vi "Laser-Main-2018-06-18.vi"() -> ()   [LabVIEW 2013]
doc: "Use this template to build a user interface event handler design pattern. Use this pattern for dialog boxes and other user interfaces. You also can create and execute user-defined events that the VI can handle the same way as user interface events."
uses:
  <vilib>/Instr/_visa.llb/VISA Configure Serial Port (Instr).vi
panel:
  out "hex integer string 2":string
  out "EnergyCommand 2":string
  in  "SetTrans 2":i16=1 min=0 max=100
  in  "OFF_Laser":bool
  out "Energy":string
  out "ReturnState":string
  in  "ShutDownSystem":bool
  out "ReturnShortState":string
  out "ShortState":string
  out "LaserState":bool[](array[boolean])
  out "hex integer string":string
  out "EnergyCommand":string
  out "HVCommand":string
  out "FreqCommand":string
  in  "SetTrans":i16=1 min=0 max=100
  in  "LaserHV":u8=20
  in  "LaserFreq":u8=60
  out "LaserEnergy uJ":dbl
  in  "ComForLaser":refnum<visa-resource-name>="COM3"
  in  "Serial Settings":T1={"baud rate"=9600, "data bits"=8, "parity"=enum."None", "stop bits"=10, "flow control"=0} {"flow control" items=["None"=0, "XON/XOFF"=1, "RTS/CTS"=2, "DTR/DSR"=4]; "stop bits" items=["1.0"=10, "1.5"=15, "2.0"=20]; "data bits" min=5 max=8 step=1; "baud rate" items=["75"=75, "110"=110, "134"=134, "150"=150, "300"=300, "600"=600, "1200"=1200, "1800"=1800, "2400"=2400, "4800"=4800, "7200"=7200, "9600"=9600, "14400"=14400, "19200"=19200, "28800"=28800, "38400"=38400, "56000"=56000, "57600"=57600, "115200"=115200, "128000"=128000, "230400"=230400]}
  in  "Stop_Laser":bool
  in  "Start_Laser":bool
  # "连接"
  # "待机"
  # "发射"
  # "内存"
  # "测能"
  # "温警"
  # "静态"
  # "操作"
  # "将激光能量设置改成激光光栅设置"
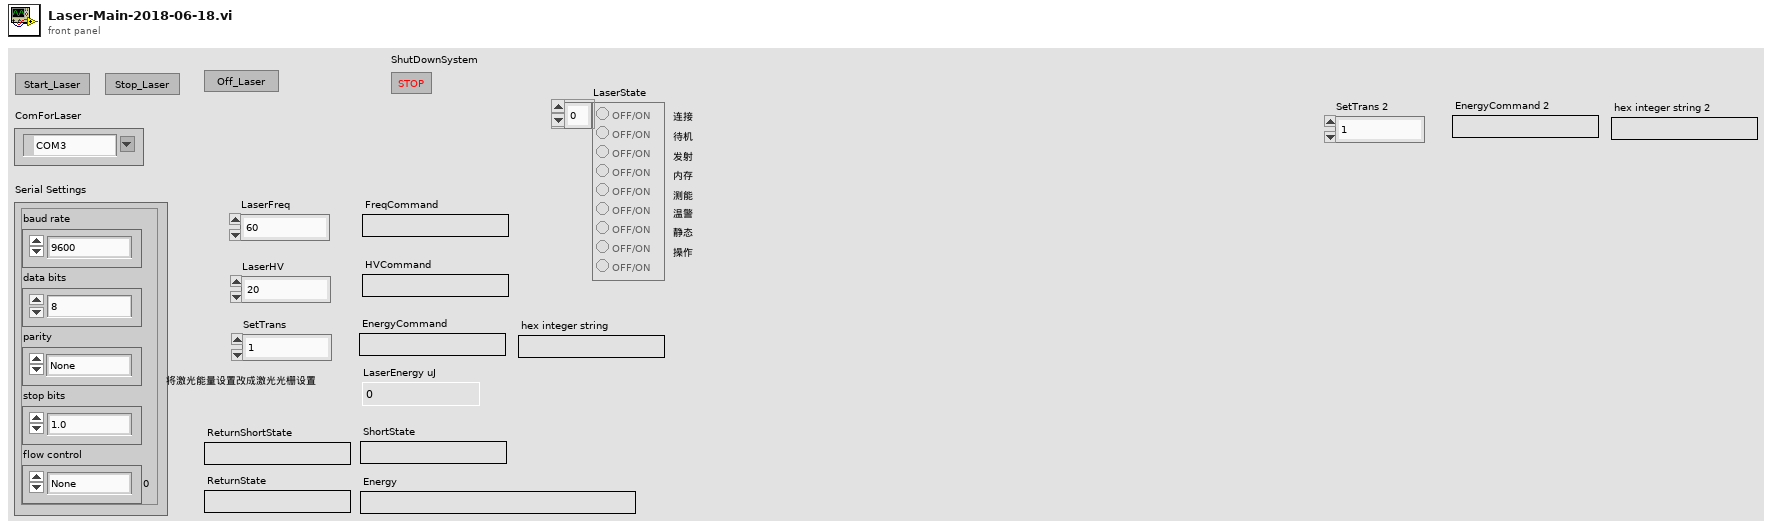
[diagram p1: front panel]
types:
  T1 = cluster{"baud rate":u32, "data bits":u16, "parity":enum16{"None", "Odd", "Even", "Mark", "Space"}, "stop bits":u16, "flow control":u16}
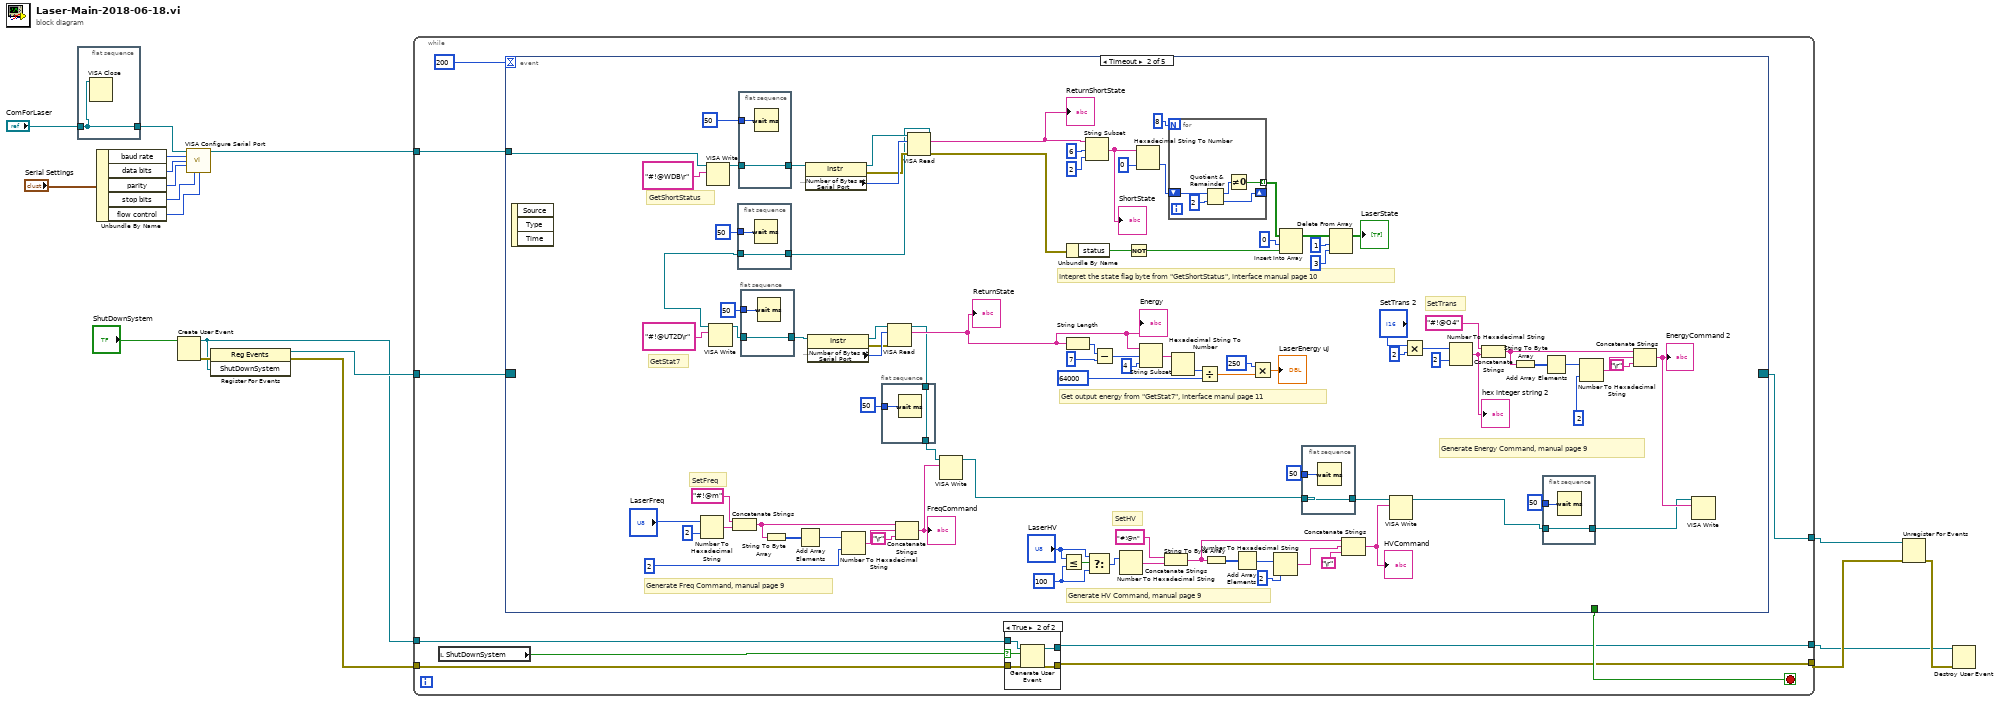
[diagram p0: block diagram]
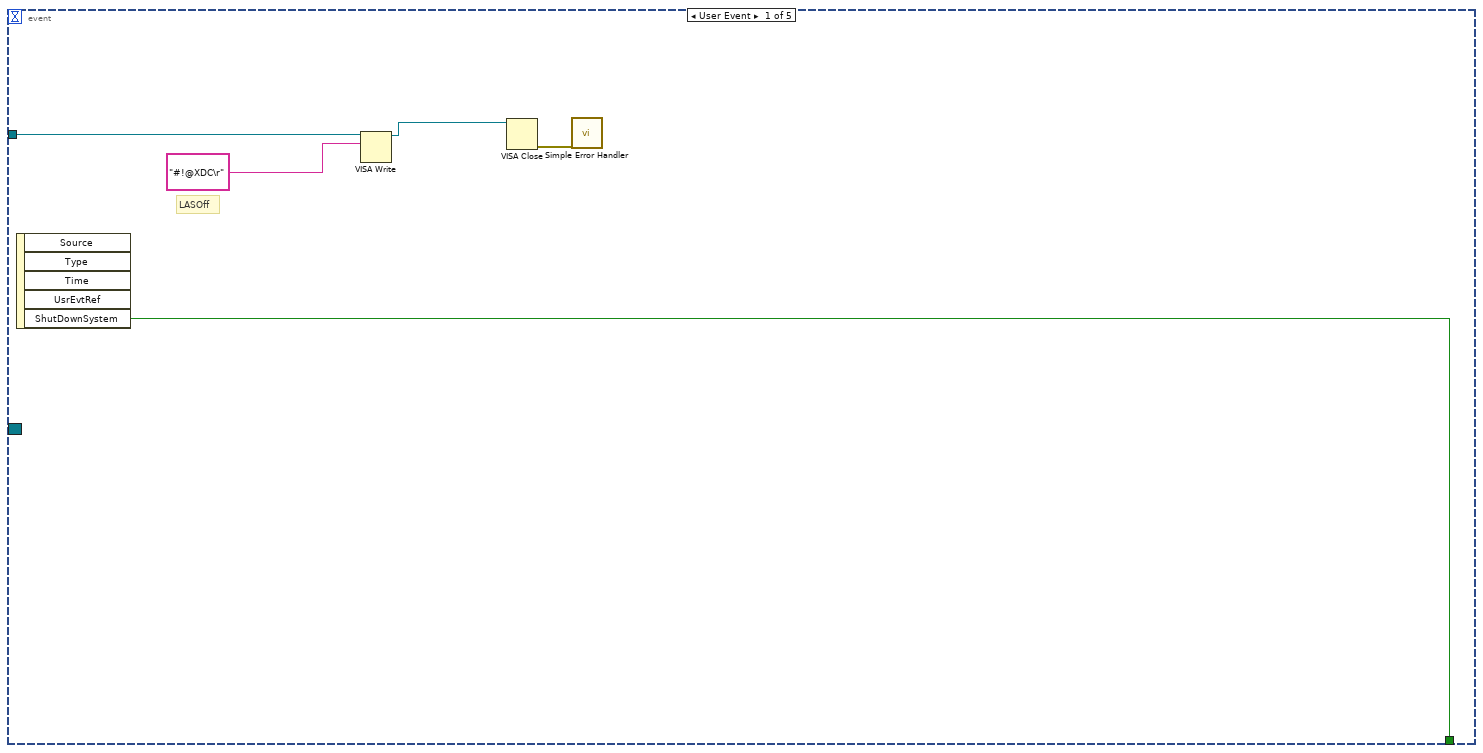
[diagram p3: hidden frame]
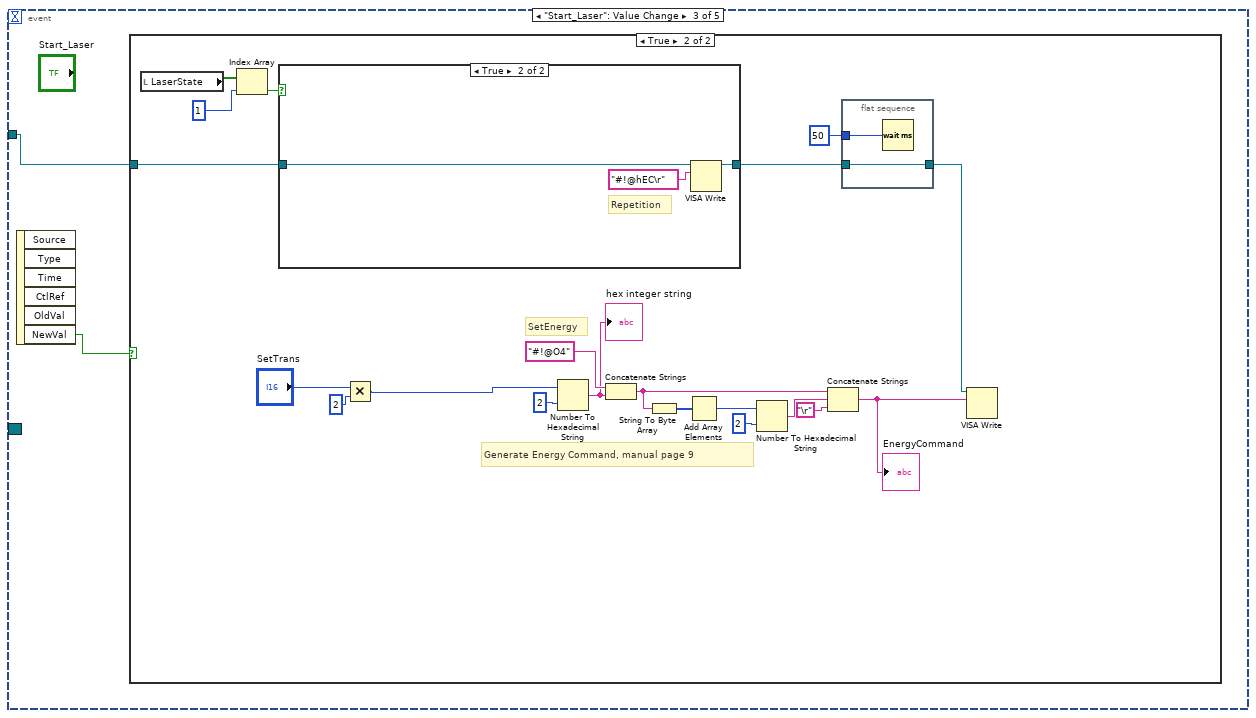
[diagram p4: hidden frame]
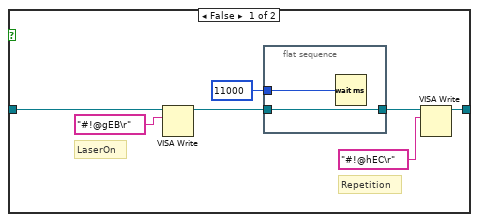
[diagram p6: hidden frame]
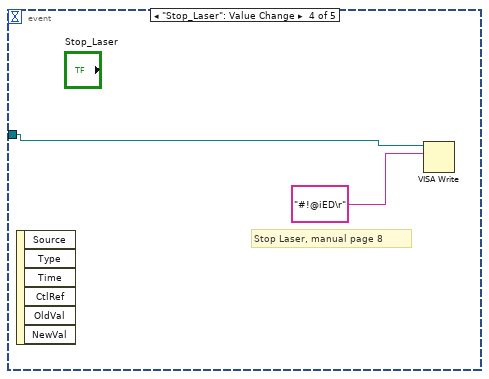
[diagram p7: hidden frame]
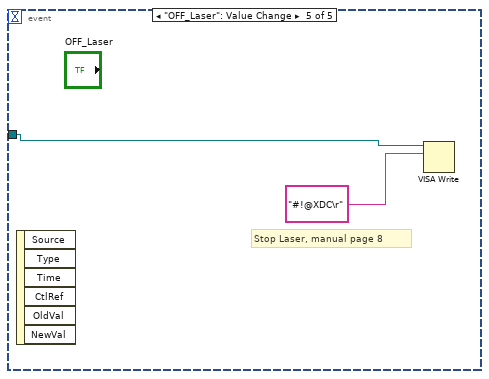
[diagram p8: hidden frame]
diagram:
  n1 = flat-sequence {
    tunnel: "ComForLaser" -> [w19]
    tunnel: [w19] -> w11
    frame #0 {
      n2 = VISA Close(VISA resource name=w19) -> ()  [unwired: 1 in, 1 out]
    }
  }
  n3 = Unbundle By Name("Serial Settings") -> ("baud rate"=w17:u32, "data bits"=w16:u16, "parity"=w15:enum16{"None", "Odd", "Even", "Mark", "Space"}, "stop bits"=w14:u16, "flow control"=w13:u16)
  n4 = Create User Event(user event datatype="ShutDownSystem") -> (user event=w5:refnum<user-event>, error out=w7:errorcluster)  [unwired: 1 in]
  n5 = call-poly "VISA Configure Serial Port"("VISA resource name"=w11, "baud rate (9600)"=w17, "data bits (8)"=w16, "parity (0:none)"=w15, "stop bits (10: 1 bit)"=w14, "flow control (0:none)"=w13) -> ("VISA resource name out"=w10:refnum<visa-resource-name>)  [unwired: 3 in, 6 out]
  n6 = register-events(error in=w7, w5) -> (reference out=w8:refnum<event-registration>, error out=w6:errorcluster)  [unwired: 1 in]
  n7 = while {
    tunnel: w10 -> [w28]
    tunnel: w8 -> [w27]
    tunnel: w6 -> [w25]
    tunnel: w5 -> [w24]
    tunnel: [w22] -> w4
    tunnel: [w21] -> w3
    tunnel: [w20] -> w1
    stop <- w23 stop-if-true
    n8 = local read "ShutDownSystem"() -> (w26:bool)
    n9 = event shown="[1] Timeout" {
      selector: w27 -> [_ _ _ _ _]
      dyn-events: [_ _ _ _ _] -> w22
      timeout: 200 -> [_ _ _ _ _]
      tunnel: w28 -> [w38 w60 w151 w186 w188]
      tunnel: [w37 _ _ _ _] -> w23
      event User Event {
        # "LASOff"
        n10 = event-data() -> ("ShutDownSystem"=w37:bool)  [unwired: 1 in, 4 out]
        n11 = VISA Write(VISA resource name=w38, write buffer="#!@XDC\r") -> (VISA resource name out=w41:refnum<visa-resource-name>)  [unwired: 1 in, 2 out]
        n12 = VISA Close(VISA resource name=w41) -> (error out=w39:errorcluster)  [unwired: 1 in]
        n13 = call <vilib>:"Simple Error Handler.vi"("error in (no error)"=w39) -> ()  [unwired: 1 in, 8 out]
      }
      event Timeout {
        w87 = u8 100 ("y")
        # "Generate Energy Command, manual page 9"
        # "SetTrans"
        # "Generate HV Command, manual page 9"
        # "Generate Freq Command, manual page 9"
        # "Get output energy from \"GetStat7\", interface manul page 11"
        # "Intepret the state flag byte from \"GetShortStatus\", interface manual page 10"
        # "SetHV"
        # "SetFreq"
        # "GetStat7"
        # "GetShortStatus"
        n14 = event-data() -> ()  [unwired: 1 in, 3 out]
        n15 = Number To Hexadecimal String(1:i16 2 ("width (-)"), 2:"LaserFreq") -> (0:w101:string)
        n16 = VISA Write(VISA resource name=w60, write buffer="#!@WDB\r") -> (VISA resource name out=w127:refnum<visa-resource-name>)  [unwired: 1 in, 2 out]
        n17 = VISA Write(VISA resource name=w92, write buffer="#!@UT2D\r") -> (VISA resource name out=w117:refnum<visa-resource-name>)  [unwired: 1 in, 2 out]
        n18 = Concatenate Strings("#!@m" ("string"), w101) -> (w97:string)
        n19 = flat-sequence {
          tunnel: [w142] -> w92
          tunnel: w93 -> [w142]
          tunnel: u32 50 ("delay before read (ms)") -> [w143]
          frame #0 {
            n20 = Wait (ms)(milliseconds to wait=w143) -> ()  [unwired: 1 out]
          }
        }
        n21 = flat-sequence {
          tunnel: w127 -> [w148]
          tunnel: [w148] -> w128
          tunnel: u32 50 ("delay before read (ms)") -> [w149]
          frame #0 {
            n22 = Wait (ms)(milliseconds to wait=w149) -> ()  [unwired: 1 out]
          }
        }
        n23 = flat-sequence {
          tunnel: w117 -> [w146]
          tunnel: [w146] -> w118
          tunnel: u32 50 ("delay before read (ms)") -> [w147]
          frame #0 {
            n24 = Wait (ms)(milliseconds to wait=w147) -> ()  [unwired: 1 out]
          }
        }
        n25 = String To Byte Array(string=w97) -> (unsigned byte array=w100:u8[])
        n26 = Add Array Elements(numeric array=w100) -> (sum=w99:u8)
        n27 = property class="Instr"(reference=w128) -> (reference out=w129:refnum<visa-resource-name>, error out=w130:errorcluster, "Serial Settings:Number of Bytes at Serial Port"=w131:u32)  [unwired: 1 in]
        n28 = property class="Instr"(reference=w118) -> (reference out=w119:refnum<visa-resource-name>, error out=w120:errorcluster, "Serial Settings:Number of Bytes at Serial Port"=w121:u32)  [unwired: 1 in]
        n29 = Number To Hexadecimal String(1:i16 2 ("width (-)"), 2:w99) -> (0:w96:string)
        n30 = flat-sequence {
          tunnel: u32 50 ("delay before read (ms)") -> [w145]
          tunnel: w59 -> [w144]
          tunnel: [w144] -> w58
          frame #0 {
            n31 = Wait (ms)(milliseconds to wait=w145) -> ()  [unwired: 1 out]
          }
        }
        n32 = VISA Read(VISA resource name=w119, byte count=w121, error in (no error)=w120) -> (VISA resource name out=w59:refnum<visa-resource-name>, read buffer=w112:string)  [unwired: 2 out]
        "ReturnState" <- w112
        "Energy" <- w112
        n33 = Concatenate Strings(w97, w96, "\r") -> (w90:string)
        "FreqCommand" <- w90
        n34 = VISA Read(VISA resource name=w129, byte count=w131, error in (no error)=w130) -> (VISA resource name out=w93:refnum<visa-resource-name>, read buffer=w125:string, error out=w72:errorcluster)  [unwired: 1 out]
        "ReturnShortState" <- w125
        n35 = VISA Write(VISA resource name=w58, write buffer=w90) -> (VISA resource name out=w76:refnum<visa-resource-name>)  [unwired: 1 in, 2 out]
        n36 = Less Or Equal?(x="LaserHV", y=w87) -> (x <= y?=w89:bool)
        n37 = Unbundle By Name(w72) -> ("status"=w71:bool)
        n38 = String Length(string=w112) -> (length=w115:i32)
        n39 = String Subset(string=w125, offset (0)=6, length (rest)=2 ("length (rest)")) -> (substring=w64:string)
        "ShortState" <- w64
        n40 = Select(t="LaserHV", s=w89, f=w87) -> (s? t:f=w78:u8)
        n41 = Subtract(x=w115, y=7) -> (x-y=w113:i32)
        n42 = Number To Hexadecimal String(2:w78) -> (0:w85:string)  [unwired: 1 in]
        n43 = Not(x=w71) -> (.not. x?=w70:bool)
        n44 = Hexadecimal String To Number(string=w64, default (0uL)=u8 0 ("default (0 U32)")) -> (number=w65:u8)  [unwired: 1 in, 1 out]
        n45 = String Subset(string=w112, offset (0)=w113, length (rest)=4) -> (substring=w110:string)
        n46 = Concatenate Strings("#!@n" ("string"), w85) -> (w81:string)
        n47 = for {
          N: 8 -> [_]
          tunnel: [w137] -> w61 mode=indexing
          shift-right: [w136] -> _
          shift-left: w65 -> [w135]
          n48 = Quotient & Remainder(x=w135, y=2) -> (x-y*floor(x/y)=w138:i32, floor(x/y)=w136:i32)
          n49 = Not Equal To 0?(x=w138) -> (x != 0?=w137:bool)
        }
        n50 = Hexadecimal String To Number(string=w110) -> (number=w109:u32)  [unwired: 2 in, 1 out]
        n51 = Divide(x=w109, y=u32 64000) -> (x/y=w107:dbl)
        n52 = String To Byte Array(string=w81) -> (unsigned byte array=w84:u8[])
        n53 = Add Array Elements(numeric array=w84) -> (sum=w83:u8)
        n54 = Multiply(x=250, y=w107) -> (x*y=→"LaserEnergy uJ":dbl)
        n55 = Number To Hexadecimal String(1:i16 2 ("width (-)"), 2:w83) -> (0:w80:string)
        n56 = Insert Into Array(array=w61, index=0, new element=w70) -> (w62:bool[])
        n57 = flat-sequence {
          tunnel: w76 -> [w140]
          tunnel: [w140] -> w75
          tunnel: u32 50 ("delay before read (ms)") -> [w141]
          frame #0 {
            n58 = Wait (ms)(milliseconds to wait=w141) -> ()  [unwired: 1 out]
          }
        }
        n59 = Delete From Array(array=w62, length=1, index=3) -> (array with subset deleted=→"LaserState":bool[])  [unwired: 1 out]
        n60 = Concatenate Strings(w81, w80, "\r") -> (w74:string)
        "HVCommand" <- w74
        n61 = VISA Write(VISA resource name=w75, write buffer=w74) -> (VISA resource name out=w43:refnum<visa-resource-name>)  [unwired: 1 in, 2 out]
        n62 = Multiply(x="SetTrans 2", y=2) -> (x*y=w57:i32)
        n63 = Number To Hexadecimal String(1:i16 2 ("width (-)"), 2:w57) -> (0:w46:string)
        "hex integer string 2" <- w46
        n64 = Concatenate Strings("#!@O4" ("string"), w46) -> (w50:string)
        n65 = String To Byte Array(string=w50) -> (unsigned byte array=w47:u8[])
        n66 = flat-sequence {
          tunnel: w43 -> [w133]
          tunnel: [w133] -> w42
          tunnel: u32 50 ("delay before read (ms)") -> [w134]
          frame #0 {
            n67 = Wait (ms)(milliseconds to wait=w134) -> ()  [unwired: 1 out]
          }
        }
        n68 = Add Array Elements(numeric array=w47) -> (sum=w48:u8)
        n69 = Number To Hexadecimal String(1:i16 2 ("width (-)"), 2:w48) -> (0:w51:string)
        n70 = Concatenate Strings(w50, w51, "\r") -> (w54:string)
        "EnergyCommand 2" <- w54
        n71 = VISA Write(VISA resource name=w42, write buffer=w54) -> ()  [unwired: 1 in, 3 out]
      }
      event "Start_Laser": Value Change {
        n72 = event-data() -> ("NewVal"=w150:bool)  [unwired: 1 in, 5 out]
        n73 = case shown="True" w150 {
          tunnel: w151 -> [_ w155]
          frame False {
          }
          frame True {
            # "Generate Energy Command, manual page 9"
            # "SetEnergy"
            n74 = local read "LaserState"() -> (w171:bool[])
            n75 = Index Array(array=w171, index=1) -> (element=w169:bool)
            n76 = case shown="True" w169 {
              tunnel: w155 -> [w175 w184]
              tunnel: [w174 w183] -> w157
              frame False {
                # "LaserOn"
                # "Repetition"
                n77 = VISA Write(VISA resource name=w175, write buffer="#!@gEB\r") -> (VISA resource name out=w178:refnum<visa-resource-name>)  [unwired: 1 in, 2 out]
                n78 = flat-sequence {
                  tunnel: w178 -> [w182]
                  tunnel: [w182] -> w176
                  tunnel: u32 11000 ("delay before read (ms)") -> [w181]
                  frame #0 {
                    n79 = Wait (ms)(milliseconds to wait=w181) -> ()  [unwired: 1 out]
                  }
                }
                n80 = VISA Write(VISA resource name=w176, write buffer="#!@hEC\r") -> (VISA resource name out=w174:refnum<visa-resource-name>)  [unwired: 1 in, 2 out]
              }
              frame True {
                # "Repetition"
                n81 = VISA Write(VISA resource name=w184, write buffer="#!@hEC\r") -> (VISA resource name out=w183:refnum<visa-resource-name>)  [unwired: 1 in, 2 out]
              }
            }
            n82 = Multiply(x="SetTrans", y=2) -> (x*y=w152:i32)
            n83 = Number To Hexadecimal String(1:i16 2 ("width (-)"), 2:w152) -> (0:w166:string)
            "hex integer string" <- w166
            n84 = Concatenate Strings("#!@O4" ("string"), w166) -> (w162:string)
            n85 = String To Byte Array(string=w162) -> (unsigned byte array=w165:u8[])
            n86 = Add Array Elements(numeric array=w165) -> (sum=w164:u8)
            n87 = Number To Hexadecimal String(1:i16 2 ("width (-)"), 2:w164) -> (0:w161:string)
            n88 = Concatenate Strings(w162, w161, "\r") -> (w158:string)
            "EnergyCommand" <- w158
            n89 = flat-sequence {
              tunnel: u32 50 ("delay before read (ms)") -> [w173]
              tunnel: w157 -> [w172]
              tunnel: [w172] -> w156
              frame #0 {
                n90 = Wait (ms)(milliseconds to wait=w173) -> ()  [unwired: 1 out]
              }
            }
            n91 = VISA Write(VISA resource name=w156, write buffer=w158) -> ()  [unwired: 1 in, 3 out]
          }
        }
      }
      event "Stop_Laser": Value Change {
        # "Stop Laser, manual page 8"
        n92 = event-data() -> ()  [unwired: 1 in, 6 out]
        n93 = VISA Write(VISA resource name=w186, write buffer="#!@iED\r") -> ()  [unwired: 1 in, 3 out]
      }
      event "OFF_Laser": Value Change {
        # "Stop Laser, manual page 8"
        n94 = event-data() -> ()  [unwired: 1 in, 6 out]
        n95 = VISA Write(VISA resource name=w188, write buffer="#!@XDC\r") -> ()  [unwired: 1 in, 3 out]
      }
    }
    n96 = case shown="True" w26 {
      selector: w26 -> [_ w34]
      tunnel: w25 -> [w30 w36]
      tunnel: w24 -> [w31 w35]
      tunnel: [w30 w33] -> w21
      tunnel: [w31 w32] -> w20
      frame False {
      }
      frame True {
        n97 = Generate User Event(user event=w35, event data cluster=w34, error in=w36) -> (user event out=w32:refnum<user-event>, error out=w33:errorcluster)  [unwired: 1 in]
      }
    }
  }
  n98 = Unregister For Events(event registration refnum=w4, error in=w3) -> (error out=w2:errorcluster)
  n99 = Destroy User Event(user event=w1, error in=w2) -> ()  [unwired: 1 out]
